vi "Get Timestamp.vi"(8 "error in":errorcluster, 11 "CAN Message in":refnum<class "CAN Message.lvclass">) -> (0 "error out":errorcluster, 2 "Time Stamp":timestamp format="%<%x %.3X>T", 3 "CAN Message out":refnum<class "CAN Message.lvclass">)   [LabVIEW 2025, in "CAN Message.lvclass"]
uses:
  CAN Message.lvclass
  CAN Message.lvclass/CAN Message.ctl
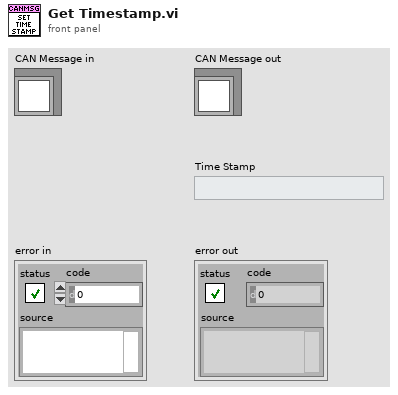
[diagram p1: front panel]
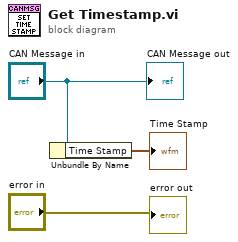
[diagram p0: block diagram]
diagram:
  n1 = Unbundle By Name("CAN Message in") -> ("Time Stamp"=→"Time Stamp":timestamp)
  "error out" <- "error in"
  "CAN Message out" <- "CAN Message in"
